vi "dSineCosine dF.vi"(7 "Freq Fitting":bool, 8 "Sampl - Ramp":dbl[](array[numeric]) format="%.5f", 9 "Coefficients":dbl[](array[numeric]) format="%.2f", 10 "Use Ramp in Model?":bool, 11 "Model In":dbl[][](array[numeric]) format="%.2f") -> (0 "V dc":dbl=0.12983305571183698 format="%.7f", 1 "d Cyc":dbl=0.12983305571183698 format="%.8f", 3 "Model Out":dbl[][](array[numeric]) format="%.6f")   [LabVIEW 2014]
uses:
  <vilib>/Analysis/baseanly.llb/A x Vector.vi
  <vilib>/Analysis/NI_AALBase.lvlib
panel:
  out "Waveform Graph":dbl[][](graph)
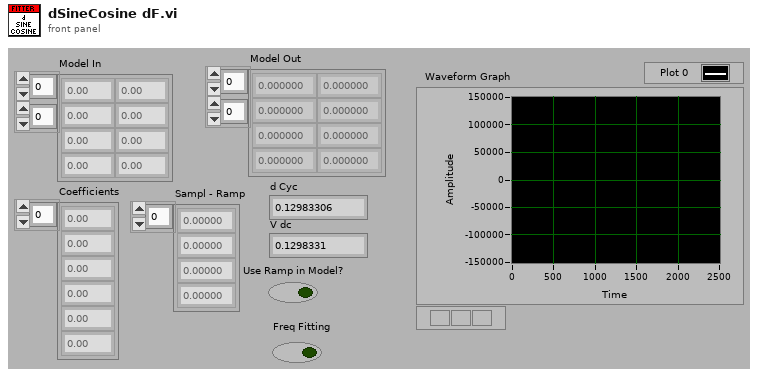
[diagram p1: front panel]
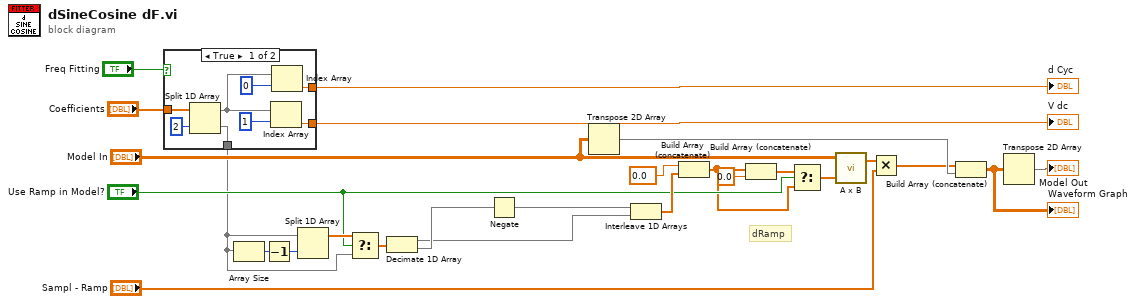
[diagram p0: block diagram]
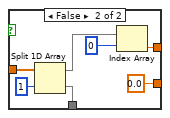
[diagram p2: hidden frame]
diagram:
  # "dRamp"
  n1 = case shown="True" "Freq Fitting" {
    tunnel: [w32 w39] -> w26
    tunnel: "Coefficients" -> [w31 w38]
    tunnel: [w29 0.0 ("Numeric")] -> w22
    tunnel: [w27 w36] -> w7
    frame True {
      n2 = Split 1D Array(array=w31, index=2) -> (first subarray=w28:dbl[], second subarray=w27:dbl[])
      n3 = Index Array(array=w28, index=1) -> (element=w29:dbl)
      n4 = Index Array(array=w28, index=0) -> (element=w32:dbl)
    }
    frame False {
      n5 = Split 1D Array(array=w38, index=1) -> (first subarray=w37:dbl[], second subarray=w36:dbl[])
      n6 = Index Array(array=w37, index=0) -> (element=w39:dbl)
    }
  }
  "d Cyc" <- w26
  "V dc" <- w22
  n7 = Array Size(array=w7) -> (size(s)=w16:i32)
  n8 = Decrement(x=w16) -> (x-1=w14:i32)
  n9 = Split 1D Array(array=w7, index=w14) -> (first subarray=w9:dbl[])  [unwired: 1 out]
  n10 = Select(t=w9, s="Use Ramp in Model?", f=w7) -> (s? t:f=w6:dbl[])
  n11 = Decimate 1D Array(w6) -> (w2:dbl[], w25:dbl[])
  n12 = Negate(x=w25) -> (-x=w1:dbl[])
  n13 = Transpose 2D Array(2D array="Model In") -> (transposed array=w19:dbl[][])
  n14 = Interleave 1D Arrays(w1, w2) -> (w21:dbl[])
  n15 = Build Array (concatenate)(0.0 ("start"), w21) -> (w4:dbl[])
  n16 = Build Array (concatenate)(w4, 0.0) -> (w11:dbl[])
  n17 = Select(t=w11, s="Use Ramp in Model?", f=w4) -> (s? t:f=w10:dbl[])
  n18 = call-poly <vilib>:"A x B.vi"("Vector"=w10, "A"="Model In") -> ("A x Vector"=w15:dbl[])  [unwired: 1 out]
  n19 = Multiply(x=w15, y="Sampl - Ramp") -> (x*y=w13:dbl[])
  n20 = Build Array (concatenate)(w13, w19) -> (w5:dbl[][])
  "Waveform Graph" <- w5
  n21 = Transpose 2D Array(2D array=w5) -> (transposed array=→"Model Out":dbl[][])
